vi "LoadCellDAQTest.vi"() -> ()   [LabVIEW 2018]
uses:
  87fd6717-2e3d-40a7-96cd-4556beea845e.vi
panel:
  in  "Valve Log Name":string="Log_Valves"
  in  "Load Cell Log Name":string="Log_LoadCell"
  in  "Sensor Log Name":string="Log_Sensors"
  in  "Log Folder":path=path "C:/LPLDocs"
  in  "Set State":T1(ring)
  out "SensorReadings":dbl[](array[numeric])
  out "Sensor State":string
  # "Load Cell DAQ Unit Test Procedure:\n\nReturn the system to the default state after each test.\n\nTest Setup:\nPower on and connect to the DAQ Box\nAttach load cell the the appropriate plug on the DAQ box, place on the ground\nSet aside a set of weights and prepare means to balance them on the load cell\n\n1) Place weights on the load cell\n        Verify that each weight detected is accurate to 2%\n        Verify that no log has been created at C:/LPLDocs\n2) Set State to Record and run test 1\n        Verify that Sensor State matches Set State at all times\n        Verify that a log file has been created in C:/LPLDocs\n        Verify that the readings contained in the log are accurate and include accurate time data in the X column\n        Verify that the data rate in the log file is <= 50Hz\n3) Set State to Record, then to Overdrive\n        Verify that Sensor State matches Set State at all times\n        Leave recording for > 5 mins, verify that  theprogram does not crash\n        Verify that the data rate in the log file starts at <=50Hz, then jumps up to >1600 Hz\n4) Set State to Record, then to Pause\n        Verify that Sensor State matches Set State at all times\n        Verify that Sensor Readings freezes once the state is Pause\n        Verify that the log file contains data which ends at the point where the state is Pause"
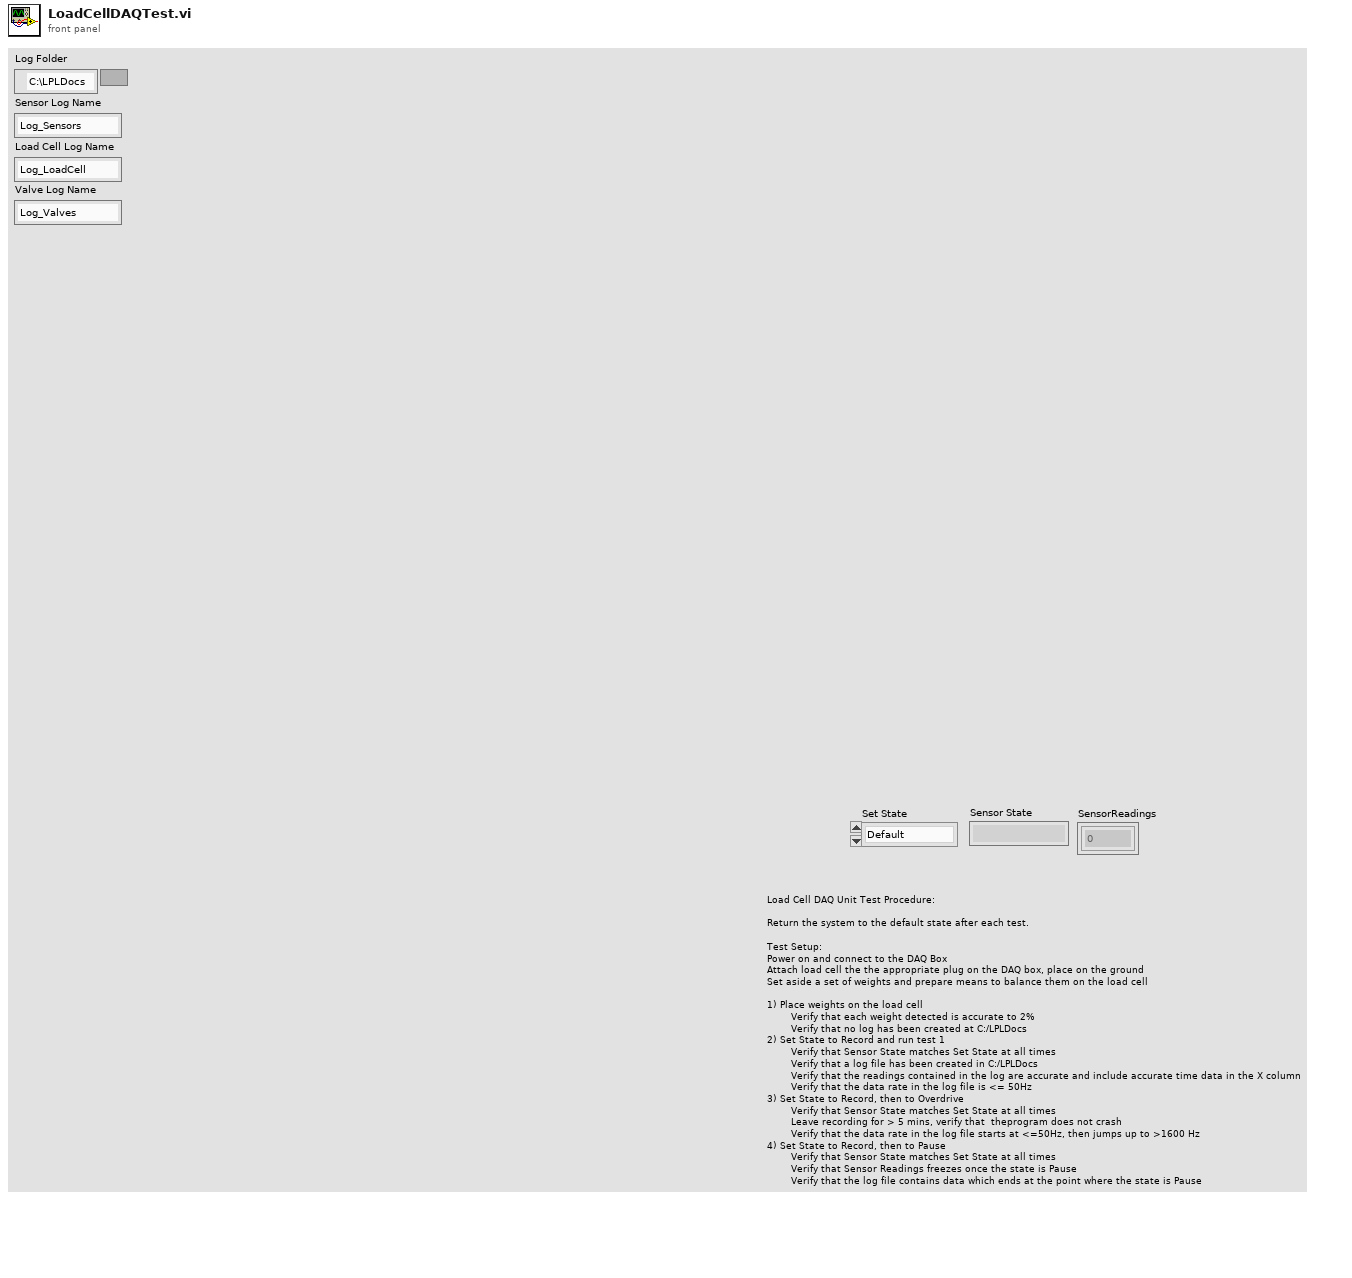
[diagram p1: front panel]
types:
  T1 = enum16{"Default", "Record", "Overdrive", "Pause"}
  T2 = enum16{"Normal", "Overdrive", "Ready for Overdrive End", "Ready for new file", "New file"}
  T3 = cluster{"SensorPath":path, "LoadCellPath":path, "ValvePath":path}
  T4 = cluster{"LoadCell Queue":refnum<queue>, "Sensor Queue":refnum<queue>, "Valve Queue":refnum<queue>}
  T5 = cluster{"Sensors":refnum<notifier>, "LoadCell":refnum<notifier>, "Fileout":refnum<notifier>, "UI":refnum<notifier>}
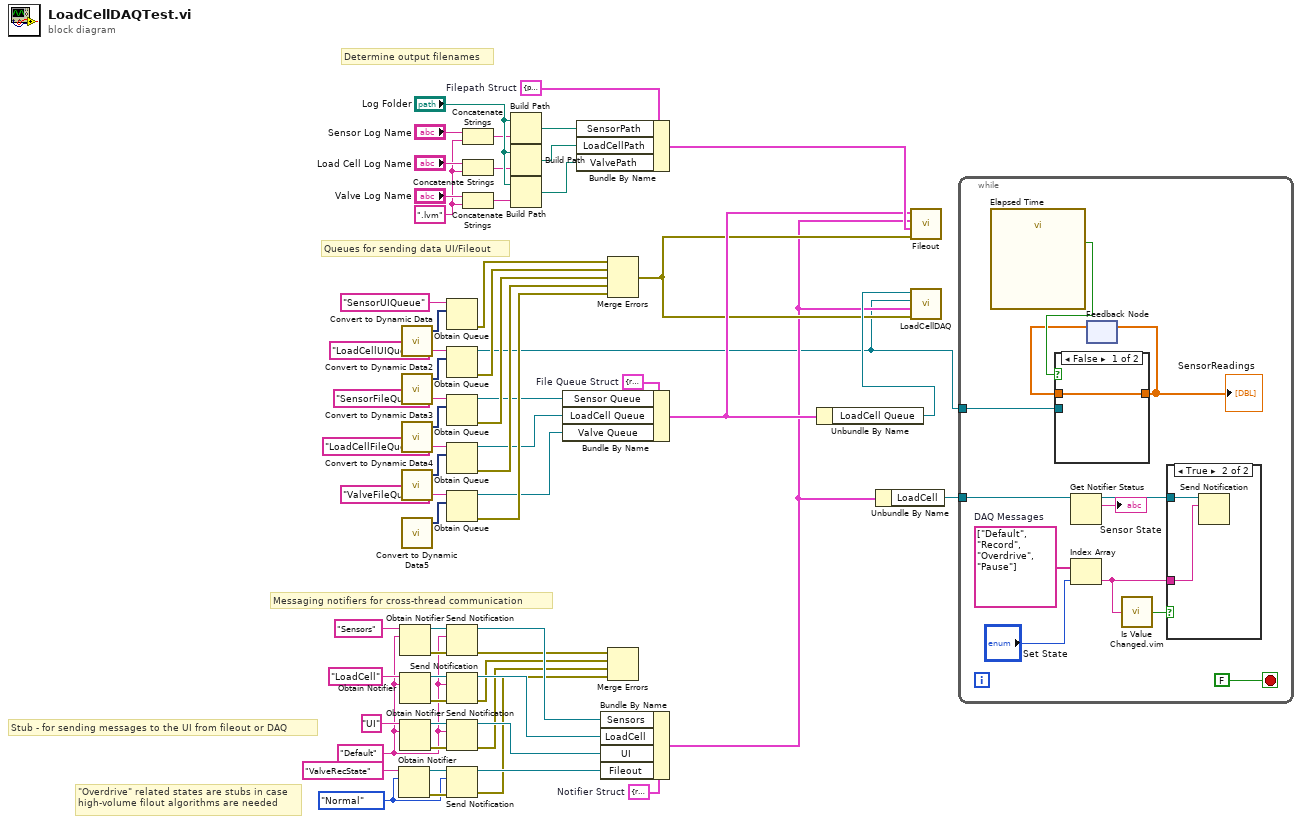
[diagram p0: block diagram]
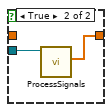
[diagram p2: hidden frame]
diagram:
  w15 = ".lvm"
  w23 = T2."Normal" ("RecState")
  w14 = T3 {"SensorPath"=path "", "LoadCellPath"=path "", "ValvePath"=path ""}  # Filepath Struct
  w10 = T4 {"LoadCell Queue"=refnum, "Sensor Queue"=refnum, "Valve Queue"=refnum}  # File Queue Struct
  w28 = T5 {"Sensors"=refnum, "LoadCell"=refnum, "Fileout"=refnum, "UI"=refnum}  # Notifier Struct
  w27 = "Default" ("RecState")
  # "Messaging notifiers for cross-thread communication"
  # "Queues for sending data UI/Fileout"
  # "Determine output filenames"
  # "Stub - for sending messages to the UI from fileout or DAQ"
  # "\"Overdrive\" related states are stubs in case\nhigh-volume filout algorithms are needed"
  n1 = Obtain Notifier(name (unnamed)="ValveRecState", notification data type=w23) -> (notifier out=w25:refnum<notifier>, error out=w24:errorcluster)  [unwired: 2 in, 1 out]
  n2 = Obtain Notifier(name (unnamed)="Sensors", notification data type=w27) -> (notifier out=w53:refnum<notifier>, error out=w52:errorcluster)  [unwired: 2 in, 1 out]
  n3 = Obtain Notifier(name (unnamed)="LoadCell", notification data type=w27) -> (notifier out=w55:refnum<notifier>, error out=w56:errorcluster)  [unwired: 2 in, 1 out]
  n4 = Obtain Notifier(name (unnamed)="UI", notification data type=w27) -> (notifier out=w57:refnum<notifier>, error out=w58:errorcluster)  [unwired: 2 in, 1 out]
  n5 = call "Convert to Dynamic Data"() -> ("Dynamic Data Type"=w42:dynamicdata)  [unwired: 4 in]
  n6 = call "Convert to Dynamic Data2"() -> ("Dynamic Data Type"=w40:dynamicdata)  [unwired: 4 in]
  n7 = call "Convert to Dynamic Data3"() -> ("Dynamic Data Type"=w38:dynamicdata)  [unwired: 4 in]
  n8 = call "Convert to Dynamic Data4"() -> ("Dynamic Data Type"=w36:dynamicdata)  [unwired: 4 in]
  n9 = call "Convert to Dynamic Data5"() -> ("Dynamic Data Type"=w34:dynamicdata)  [unwired: 4 in]
  n10 = Obtain Queue(name (unnamed)="SensorUIQueue", element data type=w42) -> (error out=w33:errorcluster)  [unwired: 3 in, 2 out]
  n11 = Obtain Queue(name (unnamed)="LoadCellUIQueue", element data type=w40) -> (queue out=w1:refnum<queue>, error out=w32:errorcluster)  [unwired: 3 in, 1 out]
  n12 = Obtain Queue(name (unnamed)="SensorFileQueue", element data type=w38) -> (queue out=w9:refnum<queue>, error out=w31:errorcluster)  [unwired: 3 in, 1 out]
  n13 = Obtain Queue(name (unnamed)="LoadCellFileQueue", element data type=w36) -> (queue out=w8:refnum<queue>, error out=w30:errorcluster)  [unwired: 3 in, 1 out]
  n14 = Obtain Queue(name (unnamed)="ValveFileQueue", element data type=w34) -> (queue out=w7:refnum<queue>, error out=w29:errorcluster)  [unwired: 3 in, 1 out]
  n15 = Send Notification(notification=w27, notifier=w53, error in (no error)=w52) -> (notifier out=w50:refnum<notifier>, error out=w46:errorcluster)
  n16 = Send Notification(notification=w27, notifier=w55, error in (no error)=w56) -> (notifier out=w49:refnum<notifier>, error out=w45:errorcluster)
  n17 = Send Notification(notification=w27, notifier=w57, error in (no error)=w58) -> (notifier out=w48:refnum<notifier>, error out=w44:errorcluster)
  n18 = Send Notification(notification=w23, notifier=w25, error in (no error)=w24) -> (notifier out=w51:refnum<notifier>, error out=w47:errorcluster)
  n19 = Concatenate Strings("Sensor Log Name", w15) -> (w18:string)
  n20 = Concatenate Strings("Load Cell Log Name", w15) -> (w17:string)
  n21 = Concatenate Strings("Valve Log Name", w15) -> (w16:string)
  n22 = Build Path(base path="Log Folder", name or relative path=w18) -> (appended path=w13:path)
  n23 = Build Path(base path="Log Folder", name or relative path=w17) -> (appended path=w12:path)
  n24 = Build Path(base path="Log Folder", name or relative path=w16) -> (appended path=w11:path)
  n25 = Bundle By Name(cluster=w10, "Sensor Queue"=w9, "LoadCell Queue"=w8, "Valve Queue"=w7) -> (w5:T4)
  n26 = Bundle By Name(cluster=w14, "SensorPath"=w13, "LoadCellPath"=w12, "ValvePath"=w11) -> (w6:T3)
  n27 = Bundle By Name(cluster=w28, "Sensors"=w50, "LoadCell"=w49, "UI"=w48, "Fileout"=w51) -> (w2:T5)
  n28 = Merge Errors(w33, w32, w31, w30, w29) -> (w3:errorcluster)
  n29 = Merge Errors(w46, w45, w44, w47) -> ()  [unwired: 1 out]
  n30 = Unbundle By Name(w5) -> ("LoadCell Queue"=w4:refnum<queue>)
  n31 = Unbundle By Name(w2) -> ("LoadCell"=w61:refnum<notifier>)
  n32 = call "Fileout.vi"("error in (no error)"=w3, "Filepaths"=w6, "Message Notifiers"=w2, "File Queues"=w5) -> ()  [unwired: 7 in, 1 out]
  n33 = call "LoadCellDAQ.vi"("error in (no error)"=w3, "Message Notifiers"=w2, "UI Queue"=w1, "Logging Queue"=w4) -> ()  [unwired: 7 in, 1 out]
  n34 = while {
    tunnel: w1 -> [w66]
    tunnel: w61 -> [w69]
    stop <- FALSE stop-if-true
    w73 = string[] ["Default", "Record", "Overdrive", "Pause"]  # DAQ Messages
    n35 = call "Elapsed Time"() -> ("Time has Elapsed"=w65:bool)  [unwired: 12 in, 7 out]
    n36 = Get Notifier Status(notifier=w69) -> (notifier out=w68:refnum<notifier>, current notification=→"Sensor State":string)  [unwired: 1 in, 3 out]
    n37 = Index Array(array=w73, index="Set State") -> (element=w70:string)
    n38 = feedback #1() -> (w63:dbl[])  [unwired: 1 in]
    n39 = case shown="False" w65 {
      tunnel: w66 -> [_ w76]
      tunnel: [w74 w75] -> w64
      tunnel: w63 -> [w74 _]
      frame False {
      }
      frame True {
        n40 = call "ProcessSignals.vi"("UI Queue"=w76) -> ("Array"=w75:dbl[])  [unwired: 9 in, 1 out]
      }
    }
    "SensorReadings" <- w64
    n41 = feedback-in #1(w64) -> ()
    n42 = call "Is Value Changed.vim"("value"=w70) -> ("changed or first call?"=w71:bool)
    n43 = case shown="True" w71 {
      tunnel: w70 -> [_ w78]
      tunnel: w68 -> [_ w77]
      frame False {
      }
      frame True {
        n44 = Send Notification(notification=w78, notifier=w77) -> ()  [unwired: 1 in, 2 out]
      }
    }
  }
